vi "SIMPS_PS_Disable.vi"(8 "error in (no error)":errorcluster) -> (0 "error out":errorcluster)   [LabVIEW 2020]
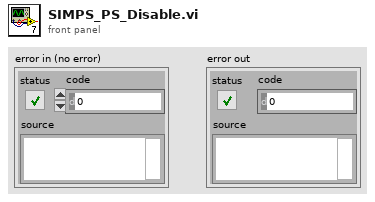
[diagram p1: front panel]
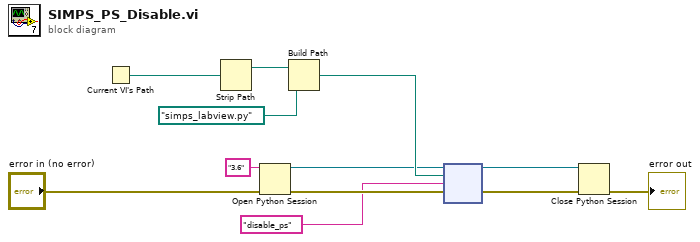
[diagram p0: block diagram]
diagram:
  n1 = Current VI's Path() -> (path=w2:path)
  n2 = Strip Path(path=w2) -> (stripped path=w1:path)  [unwired: 1 out]
  n3 = Open Python Session(python version="3.6" ("Python version"), 3:"error in (no error)") -> (session out=w4:refnum<k35>, error out=w6:errorcluster)  [unwired: 1 in]
  n4 = Build Path(base path=w1, name or relative path=path "simps_labview.py") -> (appended path=w8:path)
  n5 = node(w4, w8, "disable_ps" ("function name"), w6) -> (w10:refnum<k35>, w11:errorcluster)  [unwired: 2 in, 2 out]
  n6 = Close Python Session(session in=w10, error in=w11) -> (11:→"error out":errorcluster)
